vi "select_data.vi"() -> ()   [LabVIEW 2019]
uses:
  <vilib>/addons/database/Connection.llb/DB Tools Open Connec (Path).vi
  <vilib>/addons/database/NI_Database_API.lvlib
panel:
  in  "connection information":path
  in  "table":string
  out "data":string[][](array[string])
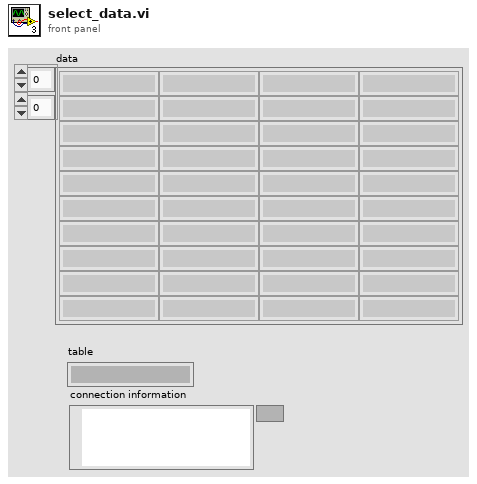
[diagram p1: front panel]
types:
  T1 = typedef "NI_Database_API.lvlib/Conn ObjectReference.ctl" = refnum<k1>
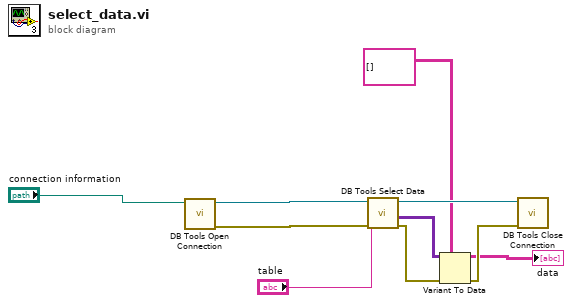
[diagram p0: block diagram]
diagram:
  n1 = call-poly <vilib>:"DB Tools Open Connection.vi"("connection information"="connection information") -> ("error out"=w3:errorcluster, "connection reference"=w10:T1)  [unwired: 7 in]
  n2 = call <vilib>:"DB Tools Select Data.vi"("error in (no error)"=w3, "table"="table", "connection reference"=w10) -> ("error out"=w7:errorcluster, "data"=w5:variant[][], "connection reference out"=w9:T1)  [unwired: 3 in]
  n3 = Variant To Data(error in=w7, type=string[][] [], Variant=w5) -> (data=→"data":string[][], error out=w8:errorcluster)
  n4 = call <vilib>:"DB Tools Close Connection.vi"("error in (no error)"=w8, "connection reference"=w9) -> ()  [unwired: 5 in, 1 out]
